vi "PythonNode_Calc_air_drop.vi"() -> ()   [LabVIEW 2019]
doc: "This example demonstrates how to call a Python function and pass clusters as arguments. It uses a python function to compute the euclidean distance between two 2D points that are represented as clusters in LabVIEW."
panel:
  out "viscosity":dbl
  out "density":dbl
  out "pressure":dbl
  in  "tau":dbl
  in  "temperature":dbl
  in  "viscosity":dbl
  in  "density":dbl
  in  "pressure":dbl
  in  "Enum":enum16{"2.7", "3.6", "3.10"}(ring)=enum."3.10"
  out "temperature":dbl format="%#_8g"
  out "error out":errorcluster
  in  "error in (no error)":errorcluster
  # "Overview: Demonstrates how to call a Python function and pass clusters as arguments.\nRequirements: Python 2.7 or 3.6 with the same bitness as LabVIEW.\nInstructions:\n1. Set the Python version to the version of Python you want to execute code in.\n2. Run the VI. You should see the euclidean distance between point 1 and point 2 in the indicator \"distance\".\n3. See comments on the block diagram of this VI and in \"ExamplePythonModule.py\" for more information about how the call python node passes arguments and handles return values."
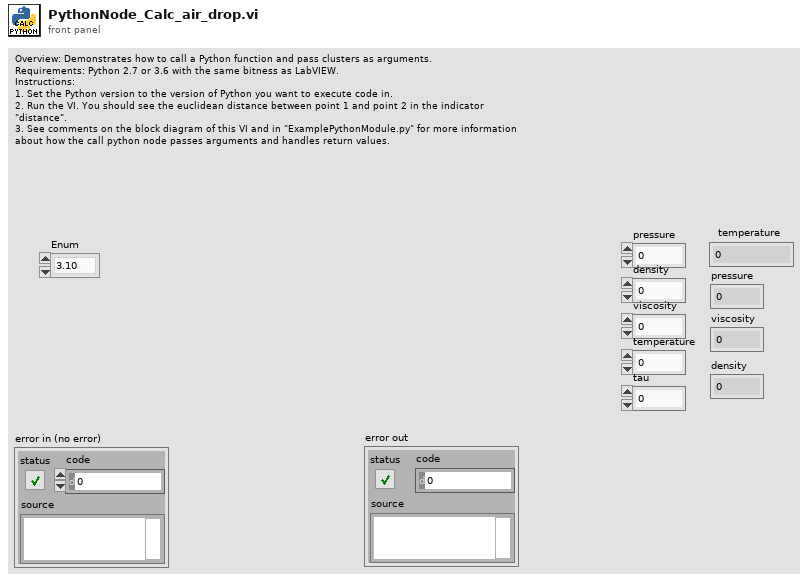
[diagram p1: front panel]
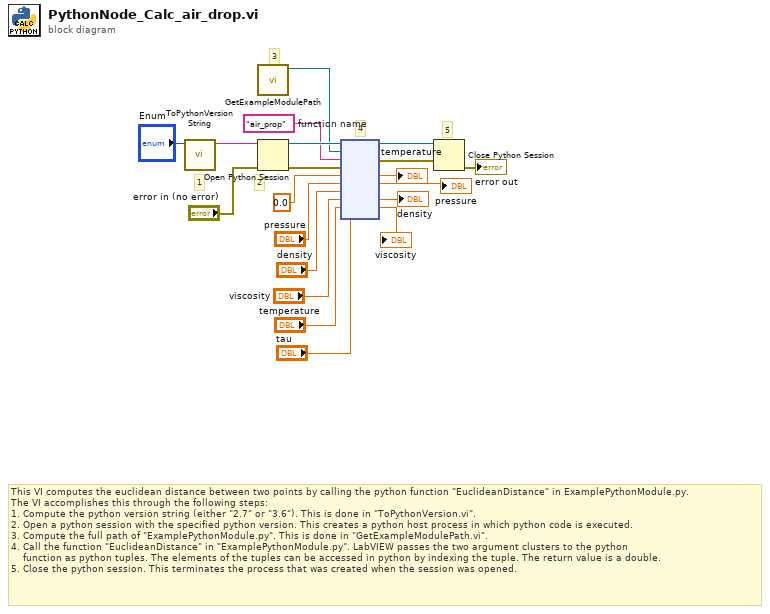
[diagram p0: block diagram]
diagram:
  w15 = "air_prop"  # function name
  # "5"
  # "4"
  # "2"
  # "3"
  # "1"
  # "This VI computes the euclidean distance between two points by calling the python function \"EuclideanDistance\" in ExamplePythonModule.py.\nThe VI accomplishes this through the following steps:\n1. Compute the python version string (either \"2.7\" or \"3.6\"). This is done in \"ToPythonVersion.vi\". \n2. Open a python session with the specified python version. This creates a python host process in which python code is executed.\n3. Compute the full path of \"ExamplePythonModule.py\". This is done in \"GetExampleModulePath.vi\".\n4. Call the function \"EuclideanDistance\" in \"ExamplePythonModule.py\". LabVIEW passes the two argument clusters to the python\n    function as python tuples. The elements of the tuples can be accessed in python by indexing the tuple. The return value is a double.\n5. Close the python session. This terminates the process that was created when the session was opened."
  n1 = call "ToPythonVersionString.vi"("Enum"="Enum") -> ("python version string"=w20:string)  [unwired: 10 in]
  n2 = call "GetExampleModulePath.vi"() -> ("module path"=w16:path)  [unwired: 11 in]
  n3 = Open Python Session(python version=w20, 3:"error in (no error)") -> (session out=w18:refnum<k35>, error out=w17:errorcluster)  [unwired: 1 in]
  n4 = node(w18, w16, w15, w17, 0.0 ("str1"), "pressure", "density", "viscosity", "temperature", "tau") -> (w14:refnum<k35>, w13:errorcluster, →"temperature":dbl, →"pressure":dbl, →"density":dbl, →"viscosity":dbl)  [unwired: 2 in, 2 out]
  n5 = Close Python Session(session in=w14, error in=w13) -> (11:→"error out":errorcluster)
